vi "Plot Mouse Wheel.vi"(6 "PlatMods":T2, 7 "Loop data in":T3={"TitleCollapse"=refnum, "MouseDownState"=enum."Idle", "RightClickCache"={"Mod"={"Ctrl"=FALSE, "Shift"=FALSE}, "CoordsStart"={"Horizontal"=0, "Vertical"=0}, "CoordsEnd"={"Horizontal"=0, "Vertical"=0}, "PlotAreaBounds"={"Left"=10, "Top"=10, "Right"=0, "Bottom"=0}, "slice"=[]}, "ZoomCache"={"SuppressedPlots"=[], "LeftAxis"={"NeedsRevert?"=FALSE, "Scale Fit"=0, "Range"={"Minimum"=0.0, "Maximum"=0.0, "Increment"=0.0, "Minor Increment"=0.0, "Start"=0.0}}, "RightAxis"={"NeedsRevert?"=FALSE, "Scale Fit"=0, "Range"={"Minimum"=0.0, "Maximum"=0.0, "Increment"=0.0, "Minor Increment"=0.0, "Start"=0.0}}, "Mod"={"Shift"=FALSE}}, "UpdateTime"=0.0, "keyboard"=refnum, "visible?"=FALSE}, 8 "error in (no error)":errorcluster, 9 "Delta":i32, 10 "Coords":T1, 11 "Refs":T13) -> (0 "error out":errorcluster, 3 "Update plot?":bool, 5 "Loop data out":T3={"TitleCollapse"=refnum, "MouseDownState"=enum."Idle", "RightClickCache"={"Mod"={"Ctrl"=FALSE, "Shift"=FALSE}, "CoordsStart"={"Horizontal"=0, "Vertical"=0}, "CoordsEnd"={"Horizontal"=0, "Vertical"=0}, "PlotAreaBounds"={"Left"=10, "Top"=10, "Right"=0, "Bottom"=0}, "slice"=[]}, "ZoomCache"={"SuppressedPlots"=[], "LeftAxis"={"NeedsRevert?"=FALSE, "Scale Fit"=0, "Range"={"Minimum"=0.0, "Maximum"=0.0, "Increment"=0.0, "Minor Increment"=0.0, "Start"=0.0}}, "RightAxis"={"NeedsRevert?"=FALSE, "Scale Fit"=0, "Range"={"Minimum"=0.0, "Maximum"=0.0, "Increment"=0.0, "Minor Increment"=0.0, "Start"=0.0}}, "Mod"={"Shift"=FALSE}}, "UpdateTime"=0.0, "keyboard"=refnum, "visible?"=FALSE})   [LabVIEW 2021, in "RocketPlot.lvlib"]
uses:
  RocketPlot.lvlib
  TypeDefs/Plot UI references.ctl
  Classes/RocketPlotHandle/RocketPlotHandle.lvclass
  <userlib>/bjustice/TipStripOOPanel/Classes/TipPanelHandle/TipPanelHandle.lvclass
  TypeDefs/Plot top row.ctl
  TypeDefs/plot while loop data.ctl
  CollapsePanel/CollapsePanel.lvclass
  TypeDefs/MouseDownState.ctl
  TypeDefs/RightClickCache.ctl
  TypeDefs/RightClickCache PlatMod.ctl
  <vilib>/Utility/miscctls.llb/LVPoint32TypeDef.ctl
  <vilib>/Utility/miscctls.llb/LVRectTypeDef.ctl
  TypeDefs/Slice average.ctl
  TypeDefs/ZoomCache.ctl
  TypeDefs/RangeCache.ctl
  <vilib>/Utility/miscctls.llb/LVRangeTypeDef.ctl
  TypeDefs/ZoomCache PlatMod.ctl
  Plot Load maker V2 - scaleread grid colors.vi
  Plot scale refnum to LUT name.vi
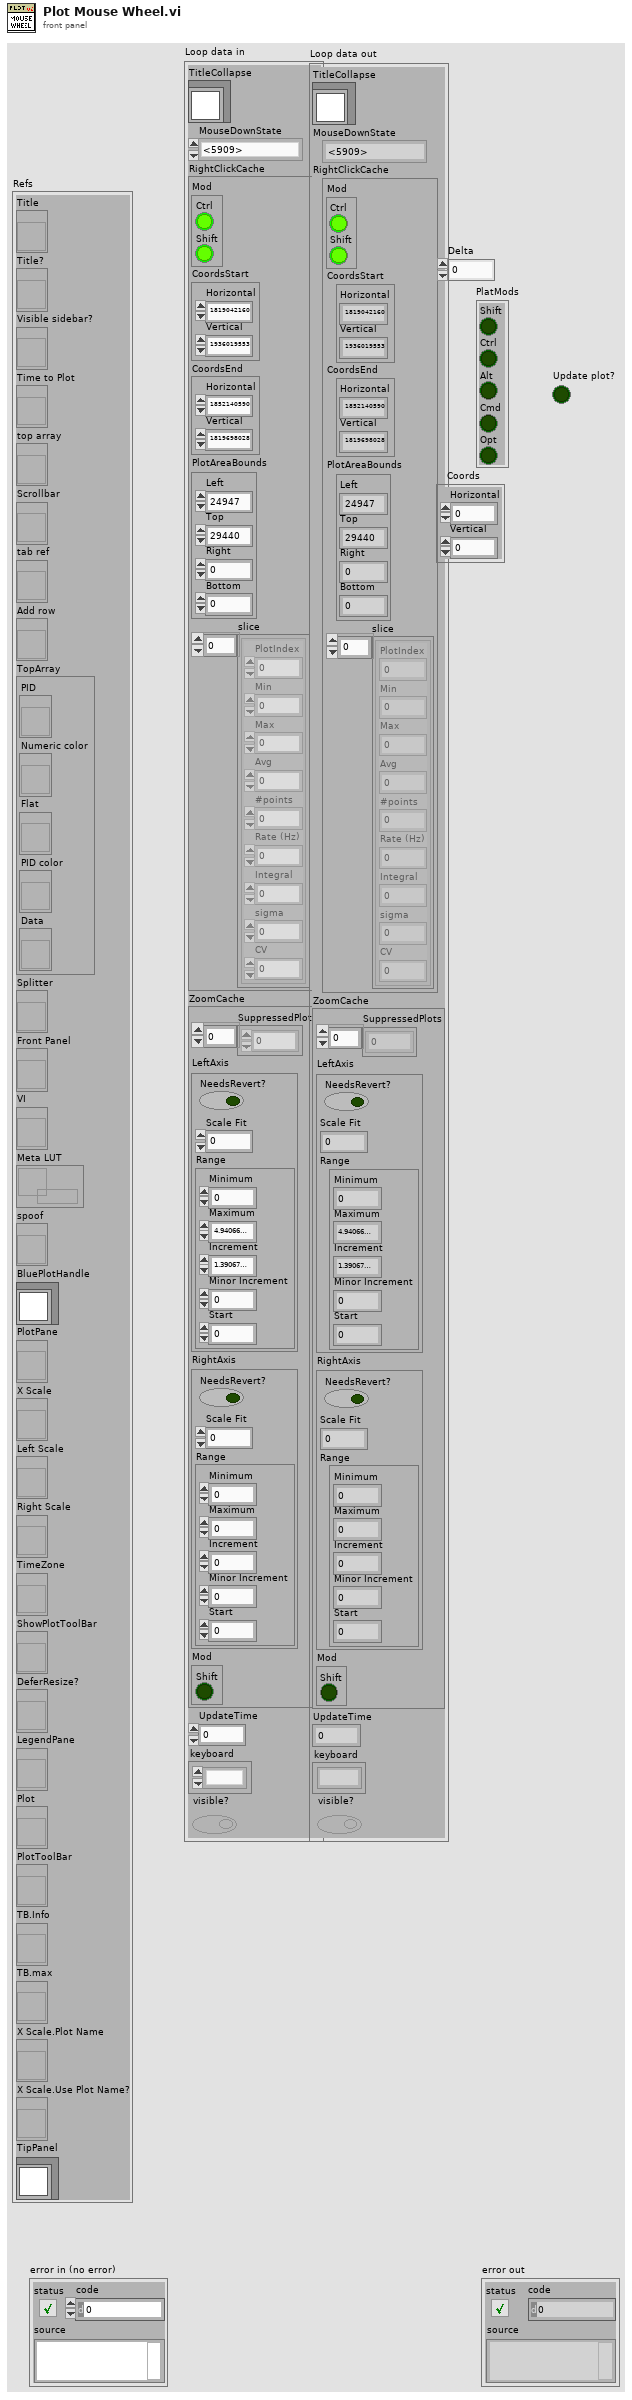
[diagram p1: front panel]
types:
  T1 = typedef "LVPoint32TypeDef.ctl" = cluster{"Horizontal":i32, "Vertical":i32}
  T2 = cluster{"Shift":bool, "Ctrl":bool, "Alt":bool, "Cmd":bool, "Opt":bool}
  T3 = typedef "RocketPlot.lvlib/plot while loop data.ctl" = cluster{"TitleCollapse":refnum<class "CollapsePanel.lvclass">, "MouseDownState":T4, "RightClickCache":T5, "ZoomCache":T9, "UpdateTime":dbl, "keyboard":refnum<k1>, "visible?":bool}
  T4 = typedef "RocketPlot.lvlib/MouseDownState.ctl" = enum16{"Idle", "Pan", "Zoom", "Zoom-Post", "RightClick"}
  T5 = typedef "RocketPlot.lvlib/RightClickCache.ctl" = cluster{"Mod":T6, "CoordsStart":T1, "CoordsEnd":T1, "PlotAreaBounds":T7, "slice":T8[]}
  T6 = typedef "RocketPlot.lvlib/RightClickCache PlatMod.ctl" = cluster{"Ctrl":bool, "Shift":bool}
  T7 = typedef "LVRectTypeDef.ctl" = cluster{"Left":i16, "Top":i16, "Right":i16, "Bottom":i16}
  T8 = typedef "RocketPlot.lvlib/Slice average.ctl" = cluster{"PlotIndex":i32, "Min":dbl, "Max":dbl, "Avg":dbl, "#points":u32, "Rate (Hz)":dbl, "Integral":dbl, "sigma":dbl, "CV":dbl}
  T9 = typedef "RocketPlot.lvlib/ZoomCache.ctl" = cluster{"SuppressedPlots":i32[], "LeftAxis":T10, "RightAxis":T10, "Mod":T12}
  T10 = typedef "RocketPlot.lvlib/RangeCache.ctl" = cluster{"NeedsRevert?":bool, "Scale Fit":u8, "Range":T11}
  T11 = typedef "LVRangeTypeDef.ctl" = cluster{"Minimum":dbl, "Maximum":dbl, "Increment":dbl, "Minor Increment":dbl, "Start":dbl}
  T12 = typedef "RocketPlot.lvlib/ZoomCache PlatMod.ctl" = cluster{"Shift":bool}
  T13 = typedef "RocketPlot.lvlib/Plot UI references.ctl" = cluster{"Title":refnum<vi>, "Title?":refnum<vi>, "Visible sidebar?":refnum<vi>, "Time to Plot":refnum<vi>, "top array":refnum<vi>, "Scrollbar":refnum<vi>, "tab ref":refnum<vi>, "Add row":refnum<vi>, "TopArray":cluster{"PID":refnum<vi>, "Numeric color":refnum<vi>, "Flat":refnum<vi>, "PID color":refnum<vi>, "Data":refnum<vi>}, "Splitter":refnum<vi>, "Front Panel":refnum<vi>, "VI":refnum<vi>, "Meta LUT":refnum<data-value>, "spoof":refnum<vi>, "BluePlotHandle":refnum<class "RocketPlotHandle.lvclass">, "PlotPane":refnum<vi>, "X Scale":refnum<vi>, "Left Scale":refnum<vi>, "Right Scale":refnum<vi>, "TimeZone":refnum<vi>, "ShowPlotToolBar":refnum<vi>, "DeferResize?":refnum<vi>, "LegendPane":refnum<vi>, "Plot":refnum<vi>, "PlotToolBar":refnum<vi>, "TB.Info":refnum<vi>, "TB.max":refnum<vi>, "X Scale.Plot Name":refnum<vi>, "X Scale.Use Plot Name?":refnum<vi>, "TipPanel":refnum<class "TipPanelHandle.lvclass">}
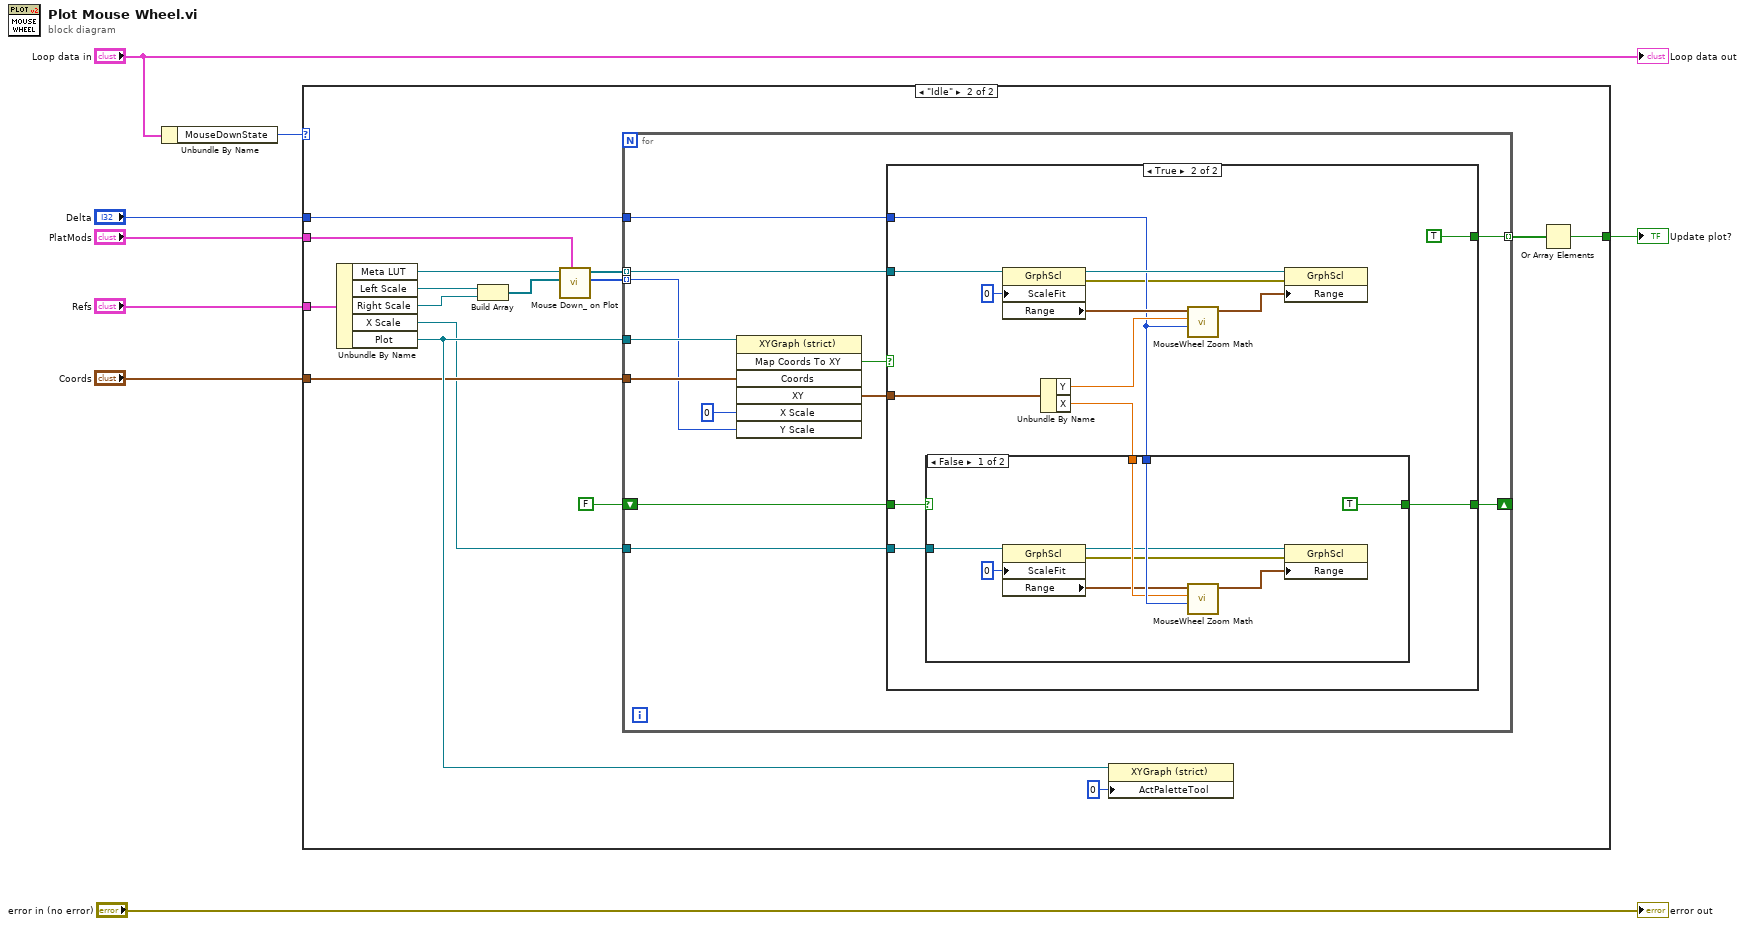
[diagram p0: block diagram]
diagram:
  n1 = Unbundle By Name("Loop data in") -> ("MouseDownState"=w5:T4)
  n2 = case shown="\"Idle\"" w5 {
    tunnel: "Refs" -> [_ w24]
    tunnel: [_ w12] -> w4
    tunnel: "PlatMods" -> [_ w23]
    tunnel: "Coords" -> [_ w15]
    tunnel: "Delta" -> [_ w11]
    frame Default {
    }
    frame "Idle" {
      n3 = Unbundle By Name(w24) -> ("Meta LUT"=w18:refnum<data-value>, "Left Scale"=w21:refnum<vi>, "Right Scale"=w20:refnum<vi>, "X Scale"=w9:refnum<vi>, "Plot"=w16:refnum<vi>)
      n4 = Build Array(w21, w20) -> (w19:refnum<vi>[])
      n5 = call "Mouse Down_ on Plot.vi"("PlatMods"=w23, "Y axes"=w19, "Meta LUT"=w18) -> ("scale index"=w14:i32[], "axes to scale"=w17:refnum<vi>[])  [unwired: 6 in, 1 out]
      n6 = for {
        tunnel: w17 -> [w36] mode=indexing
        tunnel: w16 -> [w35]
        tunnel: w15 -> [w34]
        tunnel: w14 -> [w33] mode=indexing
        tunnel: [w30] -> w13 mode=indexing
        tunnel: w11 -> [w28]
        shift-right: [w25] -> _
        shift-left: FALSE -> [w27]
        tunnel: w9 -> [w26]
        n7 = invoke class="XYGraph (strict)" method="Map Coords To XY"(reference=w35, "Coords"=w34, "X Scale"=0, "Y Scale"=w33) -> ("Map Coords To XY"=w31:bool, "XY"=w29:cluster{"X":dbl, "Y":dbl})  [unwired: 3 in, 5 out]
        n8 = case shown="True" w31 {
          tunnel: w36 -> [_ w49]
          tunnel: [_ TRUE] -> w30
          tunnel: w29 -> [_ w45]
          tunnel: w28 -> [_ w43]
          tunnel: w27 -> [w37 w39]
          tunnel: w26 -> [_ w41]
          tunnel: [w37 w38] -> w25
          frame False {
          }
          frame True {
            n9 = property class="GrphScl"(reference=w49, "ScaleFit"=u8 0 ("Scale Fit")) -> (reference out=w50:refnum<vi>, error out=w40:errorcluster, "Range"=w47:T11)  [unwired: 1 in]
            n10 = Unbundle By Name(w45) -> ("Y"=w44:dbl, "X"=w42:dbl)
            n11 = case shown="False" w39 {
              selector: w39 -> [_ w61]
              tunnel: w43 -> [w60 _]
              tunnel: w42 -> [w59 _]
              tunnel: w41 -> [w58 _]
              tunnel: [TRUE w61] -> w38
              frame False {
                n12 = property class="GrphScl"(reference=w58, "ScaleFit"=u8 0 ("Scale Fit")) -> (reference out=w54:refnum<vi>, error out=w52:errorcluster, "Range"=w55:T11)  [unwired: 1 in]
                n13 = call "MouseWheel Zoom Math.vi"("Delta"=w60, "CursorPos"=w59, "Range"=w55) -> ("Range"=w56:T11)  [unwired: 8 in]
                n14 = property class="GrphScl"(reference=w54, error in=w52, "Range"=w56) -> ()  [unwired: 2 out]
              }
              frame True {
              }
            }
            n15 = call "MouseWheel Zoom Math.vi"("Delta"=w43, "CursorPos"=w44, "Range"=w47) -> ("Range"=w46:T11)  [unwired: 8 in]
            n16 = property class="GrphScl"(reference=w50, error in=w40, "Range"=w46) -> ()  [unwired: 2 out]
          }
        }
      }
      n17 = property class="XYGraph (strict)"(reference=w16, "ActPaletteTool"=0 ("Palette:Active Tool")) -> ()  [unwired: 1 in, 2 out]
      n18 = Or Array Elements(Boolean array=w13) -> (logical OR=w12:bool)
    }
  }
  "Update plot?" <- w4
  "error out" <- "error in (no error)"
  "Loop data out" <- "Loop data in"
